vi "Pre Launch Init.vi"(11 "Nested in":refnum<class "StepMotorController.lvclass">) -> (0 "error out":errorcluster, 3 "Nested out":refnum<class "StepMotorController.lvclass">)   [LabVIEW 2020, in "StepMotorController.lvlib" / "StepMotorController.lvclass"]
doc: "(<B>Filename</B>: Actor Framework.lvlib:Actor.lvclass:Pre Launch Init.vi)\n\nDefines behavior that occurs after the Launch Nested Actor method is invoked but before the actor's Actor Core method begins running.\n\nBy default, this method does nothing. A descendant class may override it to define behavior."
uses:
  StepMotorController.lvclass
  StepMotorController.lvclass/StepMotorController.ctl
  <vilib>/ActorFramework/Actor/Actor.lvclass
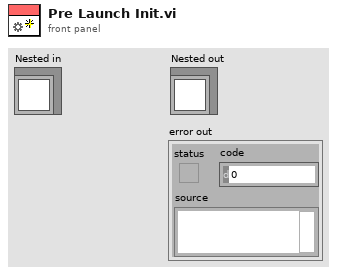
[diagram p1: front panel]
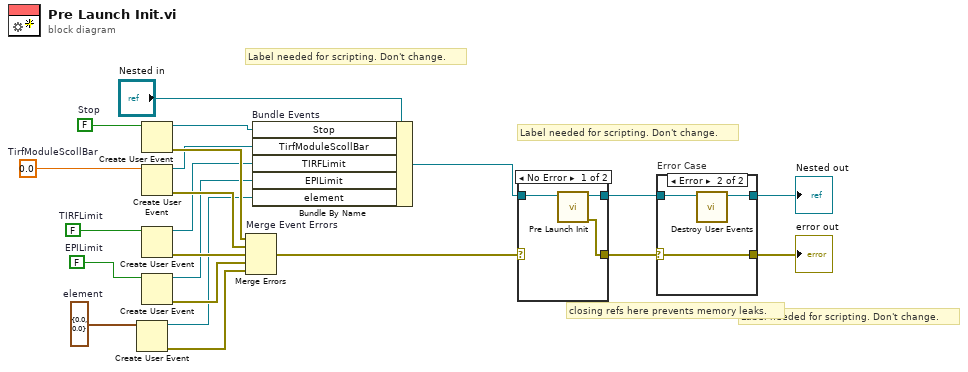
[diagram p0: block diagram]
diagram:
  w4 = cluster{"Upper limit":dbl, "Lower limit":dbl} {"Upper limit"=0.0, "Lower limit"=0.0}  # element
  w7 = FALSE  # EPILimit
  w10 = FALSE  # TIRFLimit
  w12 = 0.0  # TirfModuleScollBar
  w21 = FALSE  # Stop
  # "Label needed for scripting. Don't change."
  # "Label needed for scripting. Don't change."
  # "Label needed for scripting. Don't change."
  # "closing refs here prevents memory leaks."
  n1 = Create User Event(user event datatype=w4) -> (user event=w3:refnum<user-event>, error out=w2:errorcluster)  [unwired: 1 in]
  n2 = Create User Event(user event datatype=w21) -> (user event=w18:refnum<user-event>, error out=w20:errorcluster)  [unwired: 1 in]
  n3 = Create User Event(user event datatype=w12) -> (user event=w1:refnum<user-event>, error out=w11:errorcluster)  [unwired: 1 in]
  n4 = Create User Event(user event datatype=w10) -> (user event=w9:refnum<user-event>, error out=w8:errorcluster)  [unwired: 1 in]
  n5 = Create User Event(user event datatype=w7) -> (user event=w6:refnum<user-event>, error out=w5:errorcluster)  [unwired: 1 in]
  n6 = Merge Errors "Merge Event Errors"(w20, w11, w8, w5, w2) -> (w14:errorcluster)
  n7 = Bundle By Name "Bundle Events"(cluster="Nested in", "Stop"=w18, "TirfModuleScollBar"=w1, "TIRFLimit"=w9, "EPILimit"=w6, "element"=w3) -> (w15:refnum<class "StepMotorController.lvclass">)
  n8 = case shown="No Error" w14 {
    selector: w14 -> [_ w27]
    tunnel: [w25 w26] -> w16
    tunnel: w15 -> [w24 w26]
    tunnel: [w23 w27] -> w13
    frame No Error {
      n9 = call-parent "Pre Launch Init.vi"("Actor in"=w24) -> ("error out"=w23:errorcluster, "Actor out"=w25:refnum<class "StepMotorController.lvclass">)  [unwired: 9 in]
    }
    frame Error {
    }
  }
  n10 = case "Error Case" shown="Error" w13 {
    selector: w13 -> [w28 w32]
    tunnel: w16 -> [w29 w31]
    tunnel: [w29 w30] -> w19
    tunnel: [w28 w32] -> w17
    frame No Error {
    }
    frame Error {
      n11 = call "Destroy User Events.vi"("UI Template in"=w31) -> ("UI Template out"=w30:refnum<class "StepMotorController.lvclass">)  [unwired: 10 in]
    }
  }
  "error out" <- w17
  "Nested out" <- w19
